vi "solver.vi"(2 "Voltaje":dbl[](array[numeric]), 3 "Ec 2":dbl[](array[numeric]), 4 "Ec 1":dbl[](array[numeric])) -> (0 "y":dbl format="%#_13g", 1 "x":dbl format="%#_13g")   [LabVIEW 2014]
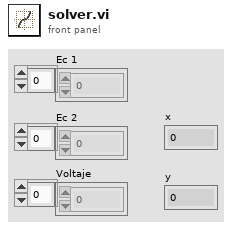
[diagram p1: front panel]
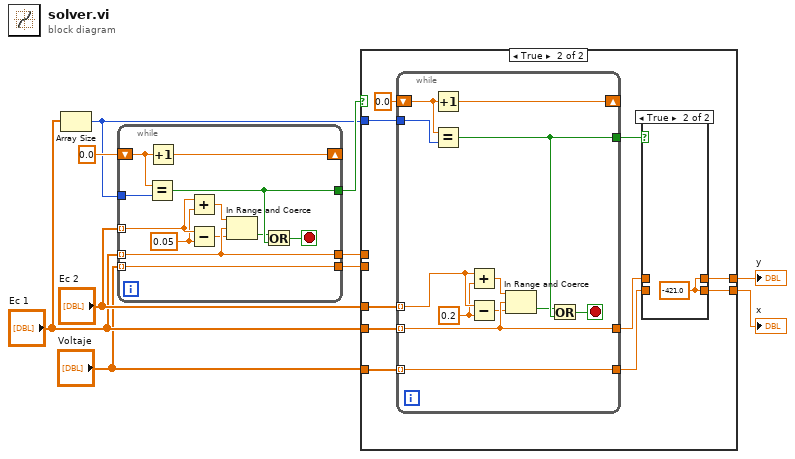
[diagram p0: block diagram]
diagram:
  n1 = Array Size(array="Ec 1") -> (size(s)=w1:i32)
  n2 = while {
    tunnel: w1 -> [w20]
    tunnel: "Ec 1" -> [w14] mode=indexing
    tunnel: "Ec 2" -> [w16] mode=indexing
    shift-right: [w22] -> _
    shift-left: 0.0 -> [w21]
    tunnel: [w14] -> w9
    tunnel: [w18] -> w7
    tunnel: "Voltaje" -> [w11] mode=indexing
    tunnel: [w11] -> w6
    stop <- w19 stop-if-true
    w15 = 0.05
    n3 = Equal?(x=w21, y=w20) -> (x = y?=w18:bool)
    n4 = Increment(x=w21) -> (x+1=w22:dbl)
    n5 = Add(x=w16, y=w15) -> (x+y=w17:dbl)
    n6 = Subtract(x=w16, y=w15) -> (x-y=w12:dbl)
    n7 = In Range and Coerce(upper limit=w17, x=w14, lower limit=w12) -> (In Range?=w13:bool)  [unwired: 1 out]
    n8 = Or(x=w13, y=w18) -> (x .or. y?=w19:bool)
  }
  n9 = case shown="True" w7 {
    tunnel: [w24 w30] -> w8
    tunnel: w9 -> [w24 _]
    tunnel: w6 -> [w23 _]
    tunnel: [w23 w29] -> w5
    tunnel: "Ec 2" -> [_ w34]
    tunnel: "Ec 1" -> [_ w33]
    tunnel: "Voltaje" -> [_ w32]
    tunnel: w1 -> [_ w28]
    frame False {
    }
    frame True {
      n10 = while {
        tunnel: w28 -> [w47]
        tunnel: w33 -> [w41] mode=indexing
        tunnel: w34 -> [w43] mode=indexing
        shift-right: [w49] -> _
        shift-left: 0.0 -> [w48]
        tunnel: [w41] -> w27
        tunnel: [w45] -> w31
        tunnel: w32 -> [w38] mode=indexing
        tunnel: [w38] -> w26
        stop <- w46 stop-if-true
        w42 = 0.2
        n11 = Increment(x=w48) -> (x+1=w49:dbl)
        n12 = Equal?(x=w48, y=w47) -> (x = y?=w45:bool)
        n13 = Add(x=w43, y=w42) -> (x+y=w44:dbl)
        n14 = Subtract(x=w43, y=w42) -> (x-y=w39:dbl)
        n15 = In Range and Coerce(upper limit=w44, x=w41, lower limit=w39) -> (In Range?=w40:bool)  [unwired: 1 out]
        n16 = Or(x=w40, y=w45) -> (x .or. y?=w46:bool)
      }
      n17 = case shown="True" w31 {
        tunnel: [w36 w37] -> w30
        tunnel: [w35 w37] -> w29
        tunnel: w27 -> [w36 _]
        tunnel: w26 -> [w35 _]
        frame False {
        }
        frame True {
          w37 = -421.0
        }
      }
    }
  }
  "y" <- w8
  "x" <- w5
